vi "Process.vi"(8 "error in (no error)":errorcluster, 10 "pound in":refnum<class "Pound.lvclass">, 11 "qbus in":refnum<class "Qbus.lvclass">) -> (0 "error out":errorcluster)   [LabVIEW 2015, in "Exposure Process.lvlib"]
doc: "Implements timer tasks that other processes register by sending Qbus messages to those processes."
uses:
  Exposure Process.lvlib
  <vilib>/addons/Qbus/Qbus.lvclass
  <vilib>/NI/Software Watchdog/Pound/Pound.lvclass
  Control_Scan Data Process.ctl
  <vilib>/addons/PointValueMap/controls/PointMap.ctl
  Control_EXP Information.ctl
  Control_File Save Setup.ctl
  Control_Enable and Path.ctl
  Control_ICM Export Setting.ctl
  <vilib>/NI/Software Watchdog/Watchdog/Watchdog.lvclass
  <vilib>/addons/PointValueMap/PointValueMap.lvlib
panel:
  out "Scan File Paths":path[](array[path])
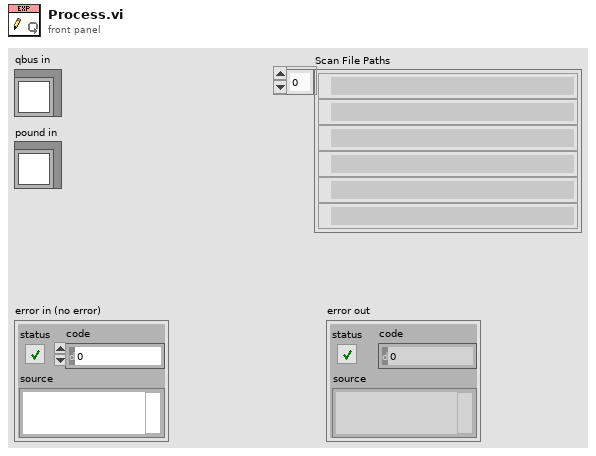
[diagram p1: front panel]
types:
  T1 = typedef "Exposure Process.lvlib/Control_Scan Data Process.ctl" = cluster{"Map - Config":T2, "Current Scan":T3, "Scan Data":variant, "Scan File Paths":path[], "Glass Data":variant, "File Save Setup":T4, "TDMS Channel Names":string[], "Combined CSV Data":string[][], "Combined Waveforms":waveform(dbl)[], "ICM Setting":T6, "RootPath":path}
  T2 = typedef "PointValueMap.lvlib/PointMap.ctl" = refnum<data-value>
  T3 = typedef "Exposure Process.lvlib/Control_EXP Information.ctl" = cluster{"Device Name":string, "Start Time":timestamp, "Path":path, "Trigger?":bool}
  T4 = typedef "Exposure Process.lvlib/Control_File Save Setup.ctl" = cluster{"Device Name":string, "Channel Names":string[], "dt":dbl, "CSV":T5, "TDMS":T5, "RAW TDMS":T5}
  T5 = typedef "Exposure Process.lvlib/Control_Enable and Path.ctl" = cluster{"Enable":bool, "Path":path}
  T6 = typedef "Exposure Process.lvlib/Control_ICM Export Setting.ctl" = cluster{"Gap":dbl, "Trigger Channel":string, "Trigger Level":dbl}
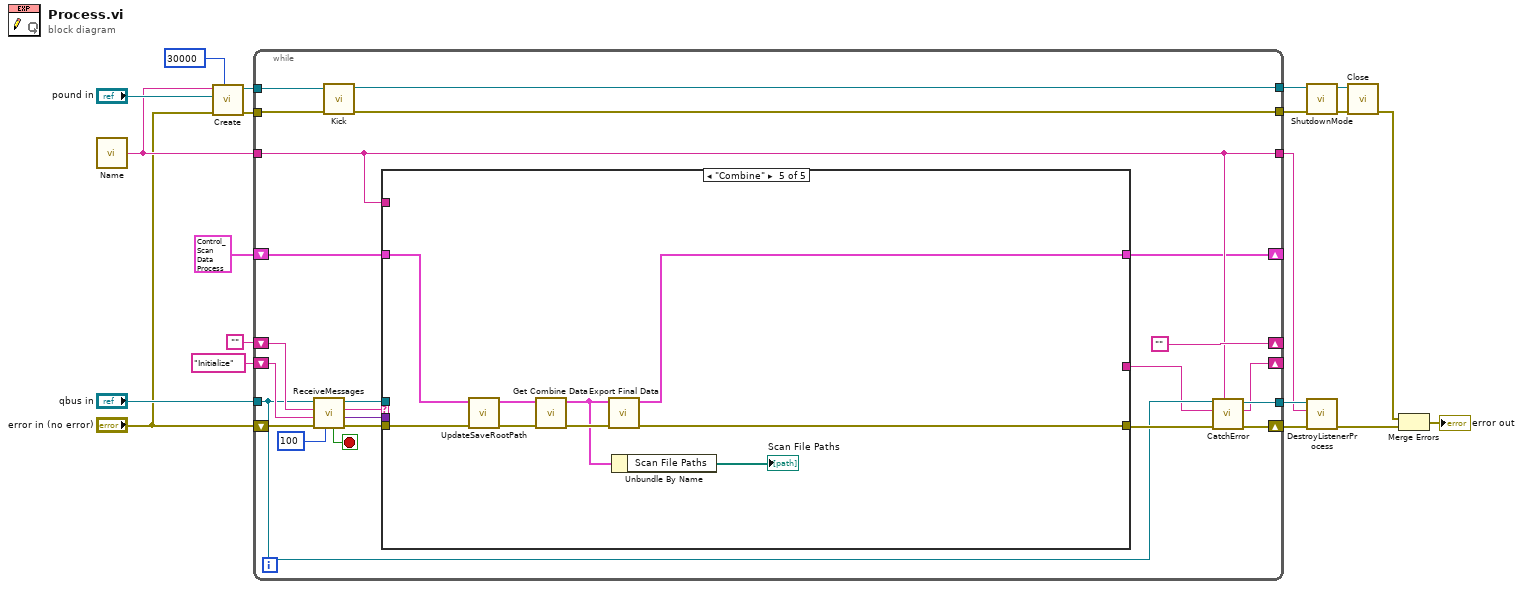
[diagram p0: block diagram]
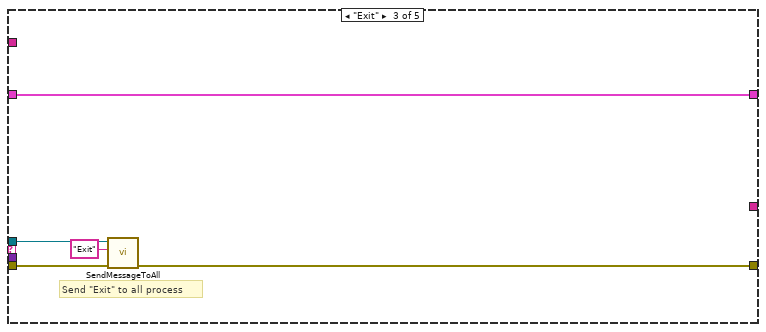
[diagram p4: hidden frame]
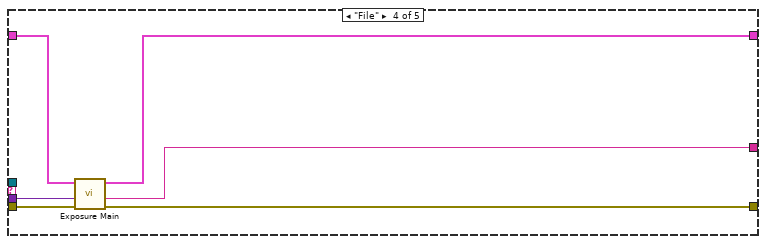
[diagram p5: hidden frame]
diagram:
  n1 = call "Name.vi"() -> ("process name"=w11:string)  [unwired: 5 in]
  n2 = call <vilib>:"Create.vi"("Execution Timeout (ms)"=u32 30000, "error in (no error)"="error in (no error)", "Pound"="pound in", "Name"=w11) -> ("error out"=w13:errorcluster, "Watchdog"=w12:refnum<data-value>)  [unwired: 6 in]
  n3 = while {
    shift-right: [""] -> _
    shift-left: "" -> [w41]
    tunnel: "qbus in" -> [w25]
    tunnel: w11 -> [w32]
    tunnel: [w34] -> w18
    tunnel: [w32] -> w17
    shift-right: [w33] -> _
    shift-left: "Initialize" -> [w36]
    tunnel: w13 -> [w30]
    tunnel: w12 -> [w29]
    tunnel: [w28] -> w6
    tunnel: [w27] -> w7
    shift-right: [w35] -> w19
    shift-left: "error in (no error)" -> [w43]
    shift-right: [w21] -> _
    shift-left: T1 {"Map - Config"=refnum, "Current Scan"={"Device Name"="", "Start Time"=timestamp(0 s since 1904-01-01), "Path"=path "", "Trigger?"=FALSE}, "Scan Data"=variant, "Scan File Paths"=[], "Glass Data"=variant, "File Save Setup"={"Device Name"="", "Channel Names"=[], "dt"=0.0, "CSV"={"Enable"=FALSE, "Path"=path ""}, "TDMS"={"Enable"=FALSE, "Path"=path ""}, "RAW TDMS"={"Enable"=FALSE, "Path"=path ""}}, "TDMS Channel Names"=[], "Combined CSV Data"=[], "Combined Waveforms"=[], "ICM Setting"={"Gap"=0.0, "Trigger Channel"="", "Trigger Level"=0.0}, "RootPath"=path ""} ("Scan Data Process") -> [w22]
    stop <- w42 stop-if-true
    n4 = call "ReceiveMessages.vi"("timeout(100)"=100, "error in (no error)"=w43, "priority action"=w36, "default action"=w41, "qbus in"=w25) -> ("error out"=w40:errorcluster, "message value"=w37:variant, "action"=w26:string, "qbus out"=w38:refnum<class "Qbus.lvclass">, "exit"=w42:bool)  [unwired: 2 in]
    n5 = call <vilib>:"Kick.vi"("error in (no error)"=w30, "Watchdog"=w29) -> ("error out"=w27:errorcluster, "Watchdog"=w28:refnum<data-value>)  [unwired: 8 in]
    n6 = case shown="\"Combine\"" w26 {
      tunnel: w40 -> [w45 w46 w52 w58 w62]
      tunnel: w38 -> [_ _ w50 _ _]
      tunnel: [w45 w46 w51 w56 w66] -> w31
      tunnel: w37 -> [_ _ _ w57 _]
      tunnel: w32 -> [_ _ _ _ _]
      tunnel: [_ _ _ w55 _] -> w23
      tunnel: w22 -> [w44 w47 w48 w54 w60]
      tunnel: [w44 w47 w48 w53 w65] -> w21
      frame "", Default {
      }
      frame "Initialize" {
        # "#reminder\nadd PVM reference"
      }
      frame "Exit" {
        # "Send \"Exit\" to all process"
        n7 = call <vilib>:"SendMessageToAll.vi"("error in (no error)"=w52, "message name"="Exit", "Qbus in"=w50) -> ("error in (no error)"=w51:errorcluster)  [unwired: 7 in, 1 out]
      }
      frame "File" {
        n8 = call "Exposure Main.vi"("error in (no error)"=w58, "Data"=w57, "Scan Data Process in"=w54) -> ("error out"=w56:errorcluster, "Combine?"=w55:string, "Scan Data Process out"=w53:T1)  [unwired: 6 in]
      }
      frame "Combine" {
        n9 = call "UpdateSaveRootPath.vi"("error in (no error)"=w62, "Scan Data Process in"=w60) -> ("error out"=w61:errorcluster, "Scan Data Process out"=w59:T1)  [unwired: 8 in]
        n10 = call "Get Combine Data.vi"("error in (no error)"=w61, "Scan Data Process in"=w59) -> ("error out"=w67:errorcluster, "Scan Data Process out"=w64:T1)  [unwired: 8 in]
        n11 = call "Export Final Data.vi"("error in (no error)"=w67, "Scan Data Process in"=w64) -> ("error out"=w66:errorcluster, "Scan Data Process out"=w65:T1)  [unwired: 8 in]
        n12 = Unbundle By Name(w64) -> ("Scan File Paths"=→"Scan File Paths":path[])
      }
    }
    n13 = call <vilib>:"CatchError.vi"("source"=w32, "error in (no error)"=w31, "next action in"=w23, "Qbus in"=w25) -> ("error out"=w35:errorcluster, "next action out"=w33:string, "Qbus out"=w34:refnum<class "Qbus.lvclass">)  [unwired: 5 in]
  }
  n14 = call <vilib>:"ShutdownMode.vi"("error in (no error)"=w7, "Watchdog"=w6) -> ("error out"=w8:errorcluster, "Watchdog"=w9:refnum<data-value>)  [unwired: 8 in]
  n15 = call <vilib>:"DestroyListenerProcess.vi"("error in (no error)"=w19, "process name"=w17, "Qbus in"=w18) -> ("error in (no error)"=w4:errorcluster)  [unwired: 7 in, 1 out]
  n16 = call <vilib>:"Close.vi"("error in (no error)"=w8, "Watchdog"=w9) -> ("error out"=w5:errorcluster)  [unwired: 9 in]
  n17 = Merge Errors(w5, w4) -> (→"error out":errorcluster)
